vi "GetAllPositions.vi"(8 "error In":errorcluster, 9 "Device Address In":i32, 10 "DeviceKey In":string, 11 "CmdLib In":refnum<k24>) -> (0 "error out":errorcluster, 1 "Device Address Out":i32, 2 "DeviceKey Out":string, 3 "CmdLib Out":refnum<k24>, 4 "Positions":i32[](array[numeric]))   [LabVIEW 2020]
uses:
  C:/GEECS/Developers Version/builds/Device builds/Picomotor8742dotNet/CmdLib.dll
  CmdLib.dll
panel:
  # "Position Motor 1"
  # "Position Motor 2"
  # "Position Motor 3"
  # "Position Motor 4"
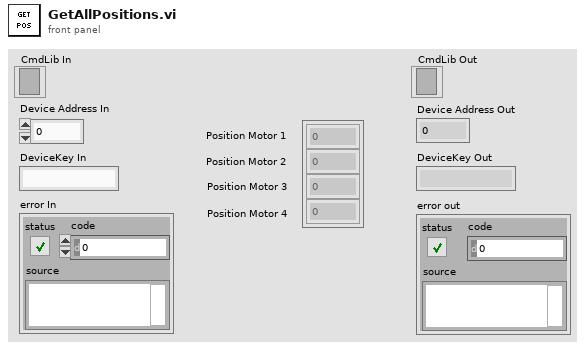
[diagram p1: front panel]
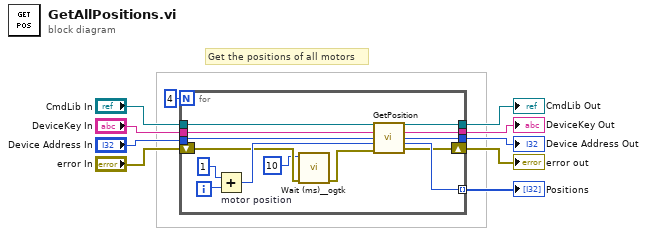
[diagram p0: block diagram]
diagram:
  # "Get the positions of all motors"
  n1 = for {
    N: 4 -> [_]
    tunnel: [w19] -> w9 mode=indexing
    tunnel: "DeviceKey In" -> [w21]
    tunnel: "CmdLib In" -> [w14]
    tunnel: [w20] -> w7
    tunnel: [w17] -> w8
    shift-right: [w18] -> w2
    shift-left: "error In" -> [w12]
    tunnel: "Device Address In" -> [w15]
    tunnel: [w16] -> w6
    i -> [w24]
    n2 = Add "motor position"(x=1 ("y"), y=w24) -> (x+y=w22:i32)
    n3 = call "Wait (ms)__ogtk.vi"("error in (no error)"=w12, "milliseconds to wait"=u32 10) -> ("error out"=w13:errorcluster)  [unwired: 8 in, 1 out]
    n4 = call "GetPosition.vi"("CmdLib In"=w14, "DeviceKey In"=w21, "Device Address In"=w15, "Motor"=w22, "error in (no error)"=w13) -> ("CmdLib Out"=w20:refnum<k24>, "DeviceKey Out"=w17:string, "Device Address Out"=w16:i32, "Position"=w19:i32, "error out"=w18:errorcluster)  [unwired: 6 in]
  }
  "Positions" <- w9
  "error out" <- w2
  "DeviceKey Out" <- w8
  "CmdLib Out" <- w7
  "Device Address Out" <- w6
